vi "Dialogue - Password Entry.vi"(9 "False Button Text (Cancel)":string="Cancel", 10 "True Button Text (OK)":string="OK", 11 "Message":string) -> (2 "PIN out":string, 3 "True Button Pressed":bool)   [LabVIEW 2015]
uses:
  UI/System Button (without mouse hover).ctl
  Utility.lvlib
  Win32 Util/Win32 Util.lvlib
  USER32.DLL
panel:
  in  "activate? (T)":bool=TRUE
  in  "z-order position":i16(ring)=2 items=["Not Topmost", "Topmost", "Top", "Bottom"]
  in  "Toggle Virtual Numpad":T1
  in  "PIN":string
  in  "False Button":T1
  in  "True Button":T1
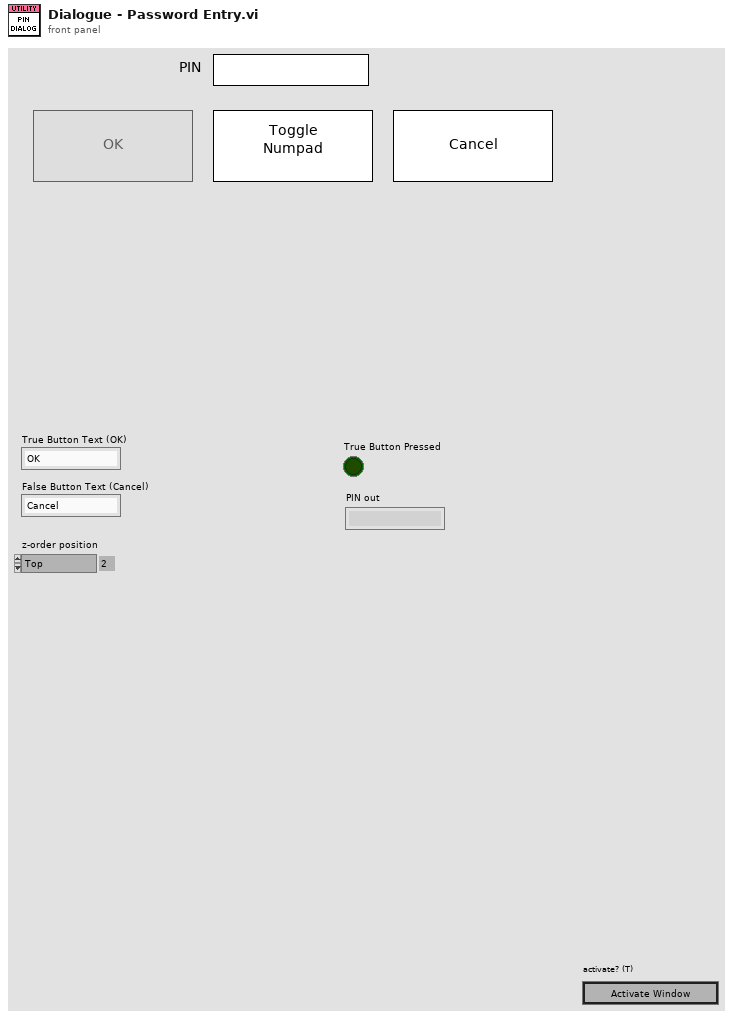
[diagram p1: front panel]
types:
  T1 = typedef "Utility.lvlib/System Button (without mouse hover).ctl" = bool
  T2 = enum8{"Enabled", "Disabled", "Disabled and Grayed Out"}
  T3 = typedef "Window Refnum" = refnum<k1>
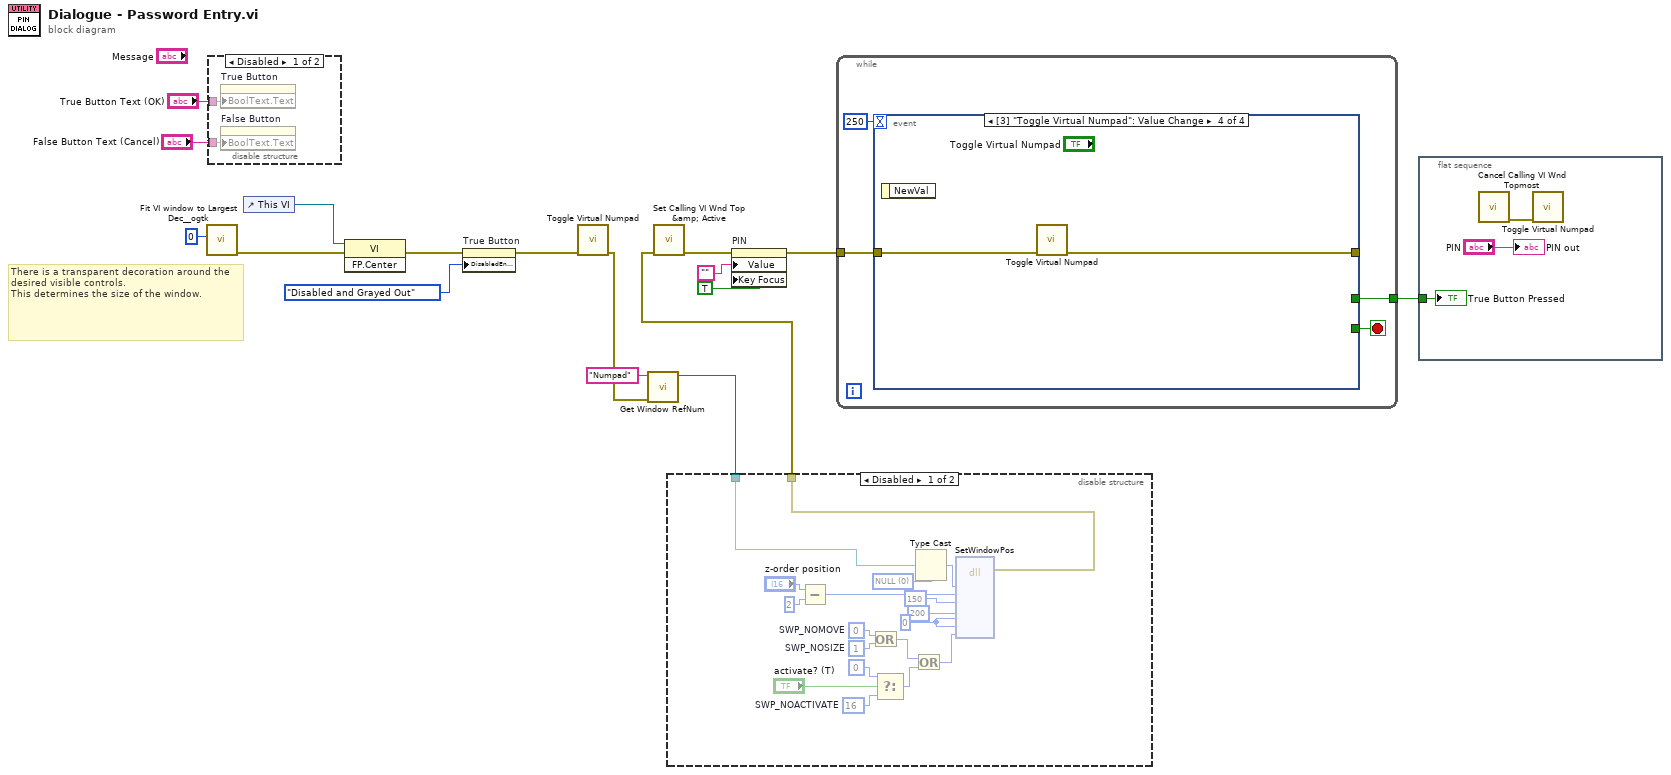
[diagram p0: block diagram]
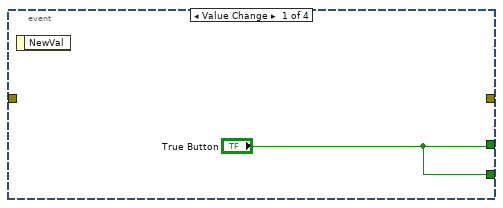
[diagram p4: hidden frame]
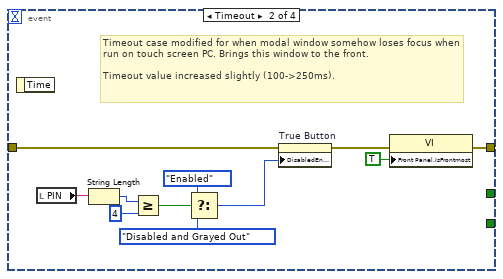
[diagram p5: hidden frame]
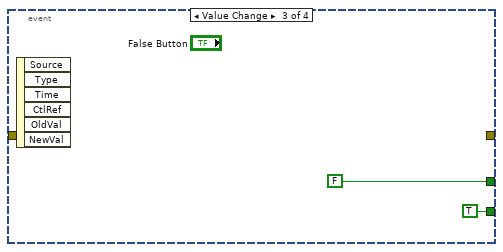
[diagram p6: hidden frame]
diagram:
  # "There is a transparent decoration around the desired visible controls.\nThis determines the size of the window."
  n1 = call <userlib>:"Fit VI window to Largest Dec__ogtk.vi"("border spacing (2 px)"=0) -> ("error out"=w15:errorcluster)  [unwired: 2 in, 4 out]
  n2 = disable-structure shown="Disabled" {
    disable-tunnel: "True Button Text (OK)" -> [w19 _]
    disable-tunnel: "False Button Text (Cancel)" -> [w18 _]
    frame Disabled {
      n3 = property on="True Button" class="Bool"("BoolText.Text"=w19) -> ()  [unwired: 2 in, 2 out]
      n4 = property on="False Button" class="Bool"("BoolText.Text"=w18) -> ()  [unwired: 2 in, 2 out]
    }
    frame Enabled {
    }
  }
  n5 = control-ref of="This VI"() -> (w1:refnum<vi>)
  n6 = invoke class="VI" method="FP.Center"(reference=w1, error in=w15) -> (error out=w4:errorcluster)  [unwired: 1 in, 2 out]
  n7 = property on="True Button" class="Bool"(error in=w4, "DisabledEnum"=T2."Disabled and Grayed Out" ("Disabled")) -> (error out=w3:errorcluster)  [unwired: 1 in, 1 out]
  n8 = call "Toggle Virtual Numpad.vi"("error in (no error)"=w3) -> ("error out"=w6:errorcluster)  [unwired: 10 in]
  n9 = call "Get Window RefNum.vi"("error in (no error)"=w6, "window name (\"\")"="Numpad" ("window name (\"\")")) -> ("window refnum (NaWR)"=w7:T3)  [unwired: 6 in, 1 out]
  n10 = disable-structure shown="Disabled" {
    disable-tunnel: w7 -> [w23 _]
    disable-tunnel: [w22 _] -> w5
    frame Disabled {
      w21 = 0
      w32 = u32 0  # SWP_NOMOVE
      w31 = u32 1  # SWP_NOSIZE
      w29 = u32 16  # SWP_NOACTIVATE
      w36 = u32 0 items=["NULL"]
      n11 = Subtract(x="z-order position", y=i16 2) -> (x-y=w33:i16)
      n12 = Or(x=w32, y=w31) -> (x .or. y?=w26:u32)
      n13 = Select(t=u32 0, s="activate? (T)", f=w29) -> (s? t:f=w27:u32)
      n14 = Or(x=w26, y=w27) -> (x .or. y?=w25:u32)
      n15 = Type Cast(type=w36, x=w23) -> (*(type *) &x=w35:u32)
      n16 = dll-call lib="USER32.DLL" fn="SetWindowPos"("hWnd"=w35, "hWndInsertAfter"=w33, "left"=150, "top"=200, "width"=w21, "height"=w21, "fuFlags"=w25) -> (error out=w22:errorcluster)  [unwired: 11 in, 1 out]
    }
    frame Enabled {
    }
  }
  n17 = call "Set Calling VI Wnd Top &amp; Active.vi"("Error In"=w5) -> ("Error Out"=w12:errorcluster)  [unwired: 10 in]
  n18 = property on="PIN" class="Str"(error in=w12, "Value"="", "Key Focus"=TRUE) -> (error out=w9:errorcluster)  [unwired: 1 in, 1 out]
  n19 = while {
    tunnel: [w41] -> w16
    tunnel: w9 -> [w40]
    stop <- w39 stop-if-true
    n20 = event shown="[3] \"Toggle Virtual Numpad\": Value Change" {
      selector: _ -> [_ _ _ _]
      dyn-events: _ -> [_ _ _ _]
      timeout: 250 -> [_ _ _ _]
      tunnel: ["True Button" _ FALSE ("True Button") _] -> w41
      tunnel: w40 -> [_ w50 _ w57]
      tunnel: [_ w44 _ w56] -> _
      tunnel: ["True Button" _ TRUE ("True Button") _] -> w39
      event Value Change {
        n21 = event-data() -> ()  [unwired: 1 in, 1 out]
      }
      event Timeout {
        # "Timeout case modified for when modal window somehow loses focus when run on touch screen PC. Brings this window to the front.\n\nTimeout value increased slightly (100->250ms)."
        n22 = event-data() -> ()  [unwired: 1 in, 1 out]
        n23 = local read "PIN"() -> (w53:string)
        n24 = String Length(string=w53) -> (length=w52:i32)
        n25 = Greater Or Equal?(x=w52, y=4) -> (x >= y?=w49:bool)
        n26 = Select(t=T2."Enabled" ("Disabled"), s=w49, f=T2."Disabled and Grayed Out" ("Disabled")) -> (s? t:f=w46:T2)
        n27 = property on="True Button" class="Bool"(error in=w50, "DisabledEnum"=w46) -> (error out=w45:errorcluster)  [unwired: 1 in, 1 out]
        n28 = property class="VI"(error in=w45, "Front Panel.IsFrontmost"=TRUE ("Front Panel Window:Is Frontmost")) -> (error out=w44:errorcluster)  [unwired: 1 in, 1 out]
      }
      event Value Change {
        n29 = event-data() -> ()  [unwired: 1 in, 6 out]
      }
      event Value Change {
        n30 = event-data() -> ()  [unwired: 1 in, 1 out]
        n31 = call "Toggle Virtual Numpad.vi"("error in (no error)"=w57) -> ("error out"=w56:errorcluster)  [unwired: 10 in]
      }
    }
  }
  n32 = flat-sequence {
    tunnel: w16 -> [w60]
    frame #0 {
      n33 = call "Cancel Calling VI Wnd Topmost.vi"() -> ("Error Out"=w58:errorcluster)  [unwired: 11 in]
      n34 = call "Toggle Virtual Numpad.vi"("error in (no error)"=w58) -> ()  [unwired: 10 in, 1 out]
      "True Button Pressed" <- w60
      "PIN out" <- "PIN"
    }
  }
